vi "Initialize.vi"(8 "error in (no error)":errorcluster, 9 "Data Cluster (for Table Headers)":variant, 10 "TableLogger Config":T1, 11 "object in":refnum<class "TableLogger_SQLite_Actor.lvclass">) -> (0 "error out":errorcluster, 3 "object out":refnum<class "TableLogger_SQLite_Actor.lvclass">)   [LabVIEW 2015, in "TableLogger_SQLite_Actor.lvlib" / "TableLogger_SQLite_Actor.lvclass"]
uses:
  TableLogger_SQLite_Actor.lvclass
  TableLogger_Actor/TableLoggerConfig.ctl
  TableLogger_Actor/TableLoggerTypes.ctl
  TableLogger_SQLite_Actor.lvclass/TableLogger_SQLite_Actor.ctl
  <vilib>/drjdpowell/SQLite Library/SQL Connection/Open (path).vi
  <vilib>/drjdpowell/SQLite Library/SQL Connection/Open (string).vi
  <userlib>/_OpenG.lib/file/file.llb/Strip Path - Traditional__ogtk.vi
  <vilib>/AdvancedString/Path To Command Line String.vi
  <vilib>/drjdpowell/SQLite Library/SQL Connection/Execute SQL (No results).vi
  <vilib>/drjdpowell/SQLite Library/SQL Connection/Connection.lvclass
  <vilib>/drjdpowell/SQLite Library/SQLite.lvlib
  TableLogger_Actor/TableLogger_Actor/TableLogger_Actor.lvclass
  TableLogger_Actor/TableLogger_Actor.lvlib
panel:
  # "Connector Pane"
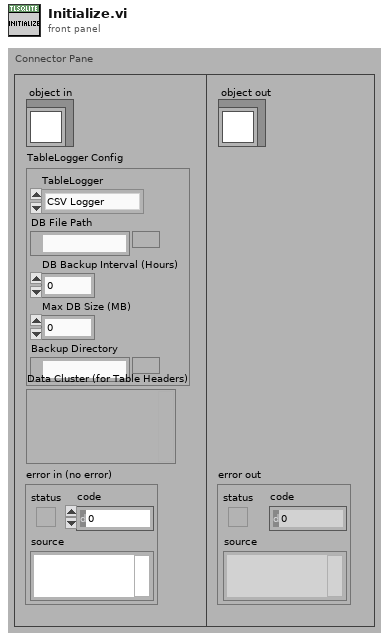
[diagram p1: front panel]
types:
  T1 = typedef "TableLogger_Actor.lvlib/TableLoggerConfig.ctl" = cluster{"TableLogger":T2, "DB File Path":path, "DB Backup Interval (Hours)":i32, "Max DB Size (MB)":i32, "Backup Directory":path}
  T2 = typedef "TableLogger_Actor.lvlib/TableLoggerTypes.ctl" = enum16{"CSV Logger", "SQLite Logger"}
  T3 = typedef "Type Descriptor Enumeration__ogtk.ctl" = enum8{"<Null>", "I8", "I16", "I32", "I64", "U8", "U16", "U32", "U64", "SGL", "DBL", "EXT", "CSG", "CDB", "CXT", "0x0F", "0x10", "0x11", "0x12", "0x13", "0x14", "Enum U8", "Enum U16", "Enum U32", "Enum U64", "SGL PQ", "DBL PQ", "EXT PQ", "CSG PQ", "CDB PQ", "CXT PQ", "0x1F", "0x20", "Boolean", "0x22", "0x23", "0x24", "0x25", "0x26", "0x27", "0x28", "0x29", "0x2A", "0x2B", "0x2C", "0x2D", "0x2E", "0x2F", "String", "0x31", "Path", "Pict", "0x34", "0x35", "0x36", "DAQ", "0x38", "0x39", "0x3A", "0x3B", "0x3C", "0x3D", "0x3E", "0x3F", "Array", "0x41", "0x42", "0x43", "0x44", "0x45", "0x46", "0x47", "0x48", "0x49", "0x4A", "0x4B", "0x4C", "0x4D", "0x4E", "0x4F", "Cluster", "0x51", "0x52", "Variant", "Waveform", "0x55", "0x56", "0x57", "0x58", "0x59", "0x5A", "0x5B", "0x5C", "0x5D", "0x5E", "0x5F", "0x60", "0x61", "0x62", "0x63", "0x64", "0x65", "0x66", "0x67", "0x68", "0x69", "0x6A", "0x6B", "0x6C", "0x6D", "0x6E", "0x6F", "Refnum"}
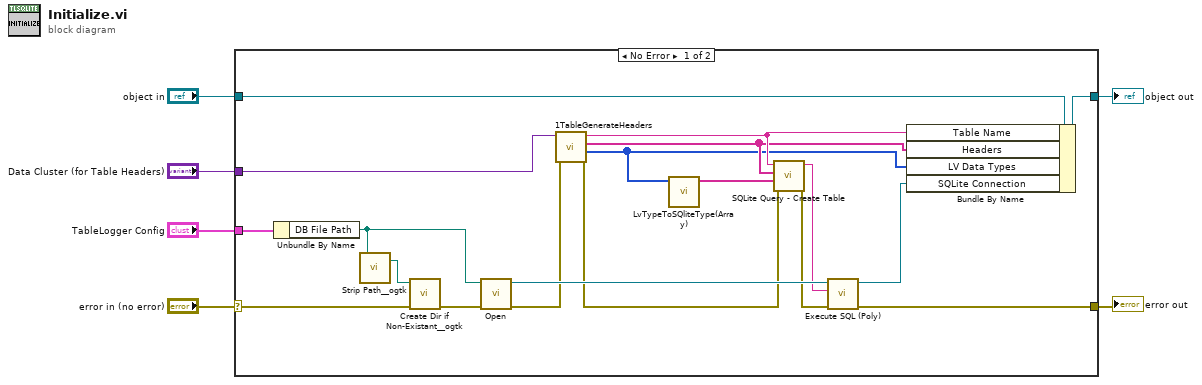
[diagram p0: block diagram]
diagram:
  n1 = case shown="No Error" "error in (no error)" {
    selector: "error in (no error)" -> [w25 w27]
    tunnel: [w20 w27] -> w5
    tunnel: [w24 w26] -> w4
    tunnel: "object in" -> [w23 w26]
    tunnel: "TableLogger Config" -> [w10 _]
    tunnel: "Data Cluster (for Table Headers)" -> [w19 _]
    frame No Error {
      n2 = Unbundle By Name(w10) -> ("DB File Path"=w9:path)
      n3 = call-poly <userlib>:"Strip Path__ogtk.vi"("path"=w9) -> ("stripped path"=w7:path)  [unwired: 1 out]
      n4 = call <userlib>:"Create Dir if Non-Existant__ogtk.vi"("error in (no error)"=w25, "Directory Path"=w7) -> ("error out"=w8:errorcluster)  [unwired: 7 in, 2 out]
      n5 = call-poly <vilib>:"Open.vi"("error in (no error)"=w8, "db file"=w9) -> ("error out"=w18:errorcluster, "SQLite Connection"=w22:refnum<class "Connection.lvclass">)  [unwired: 8 in]
      n6 = call "1TableGenerateHeaders.vi"("error in (no error)"=w18, "Cluster Variant"=w19) -> ("error out"=w17:errorcluster, "LV Data Types"=w12:T3[], "Headers"=w13:string[], "Table Name"=w14:string)  [unwired: 6 in]
      n7 = call "LvTypeToSQliteType(Array).vi"("Type Descriptor Enumeration"=w12) -> ("String"=w11:string[])  [unwired: 10 in]
      n8 = call "SQLite Query - Create Table.vi"("error in"=w17, "Table Col SQL Data Types"=w11, "Table Headers"=w13, "Table Name"=w14) -> ("error out"=w15:errorcluster, "SQLite Query"=w16:string)  [unwired: 6 in]
      n9 = call-poly <vilib>:"Execute SQL (Poly).vi"("error in (no error)"=w15, "SQL"=w16, "SQLite Connection in"=w22) -> ("error out"=w20:errorcluster, "SQLite Connection"=w21:refnum<class "Connection.lvclass">)  [unwired: 7 in]
      n10 = Bundle By Name(cluster=w23, "Table Name"=w14, "Headers"=w13, "LV Data Types"=w12, "SQLite Connection"=w21) -> (w24:refnum<class "TableLogger_SQLite_Actor.lvclass">)
    }
    frame Error {
    }
  }
  "error out" <- w5
  "object out" <- w4
